vi "Read Message.vi"(8 "error in (no error)":errorcluster, 10 "Bytes to read":i32, 11 "TCP Listener in":refnum<class "TCP Listener.lvclass">) -> (0 "error out":errorcluster, 2 "Message string":string, 3 "TCP Listener out":refnum<class "TCP Listener.lvclass">)   [LabVIEW 2026, in "TALOS.lvlib" / "TCP Listener.lvlib" / "TCP Listener.lvclass"]
uses:
  TCP Listener.lvclass
  TCP Listener.lvclass/TCP Listener.ctl
  Support VIs/Global Constants.vi
  TALOS.lvlib
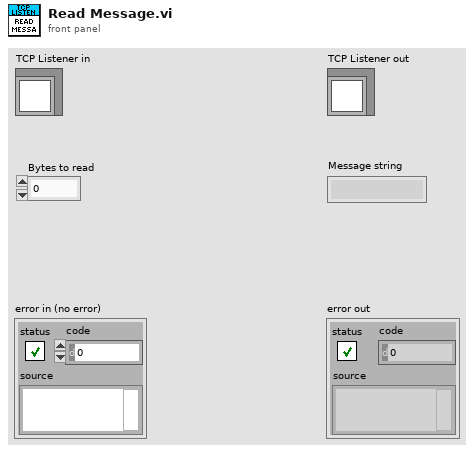
[diagram p1: front panel]
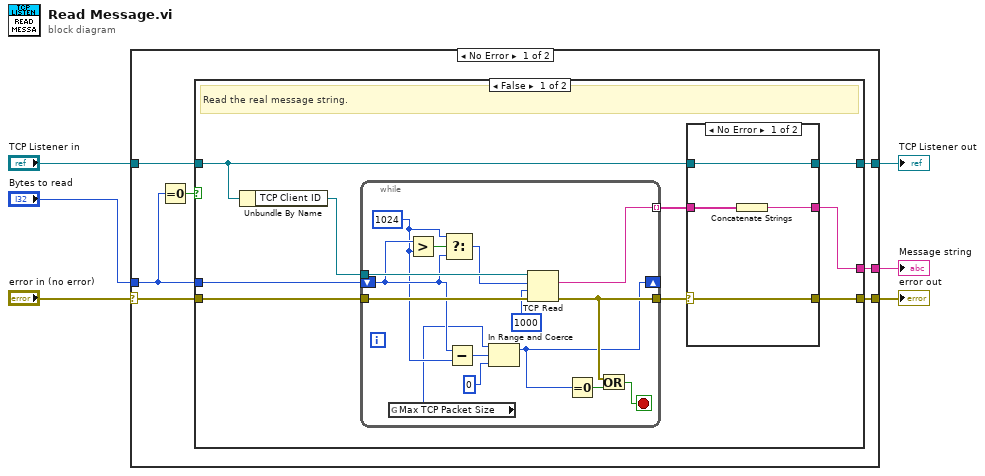
[diagram p0: block diagram]
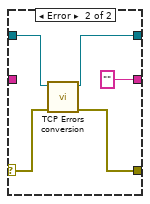
[diagram p2: hidden frame]
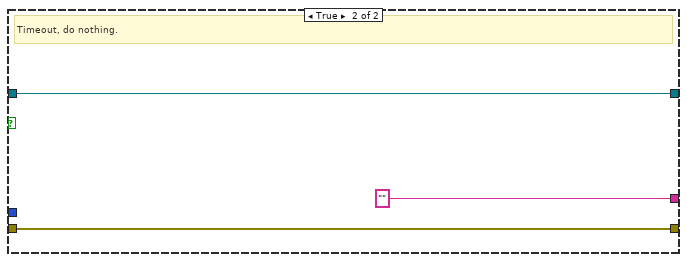
[diagram p3: hidden frame]
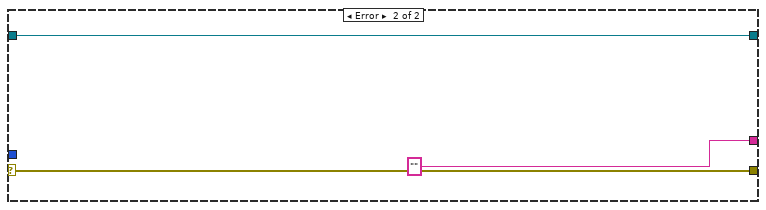
[diagram p4: hidden frame]
diagram:
  n1 = case shown="No Error" "error in (no error)" {
    selector: "error in (no error)" -> [w13 w52]
    tunnel: [w10 w52] -> w5
    tunnel: [w11 w51] -> w3
    tunnel: "TCP Listener in" -> [w12 w51]
    tunnel: "Bytes to read" -> [w7 _]
    tunnel: [w9 ""] -> w1
    frame No Error {
      n2 = Equal To 0?(x=w7) -> (x = 0?=w8:bool)
      n3 = case shown="False" w8 {
        tunnel: w7 -> [w21 _]
        tunnel: w13 -> [w20 w47]
        tunnel: w12 -> [w19 w49]
        tunnel: [w16 w49] -> w11
        tunnel: [w15 w47] -> w10
        tunnel: [w14 "" ("data out")] -> w9
        frame False {
          # "Read the real message string."
          n4 = Unbundle By Name(w19) -> ("TCP Client ID"=w22:refnum<k5>)
          n5 = while {
            tunnel: w22 -> [w37]
            tunnel: [w35] -> w17 mode=indexing
            tunnel: w20 -> [w36]
            tunnel: [w25] -> w18
            shift-right: [w24] -> _
            shift-left: w21 -> [w31]
            stop <- w27 stop-if-true
            w30 = 1024 ("timeout ms (25000)")
            n6 = global read "Global Constants.vi" "Max TCP Packet Size"() -> (w23:i32)
            n7 = Greater?(x=w31, y=w30) -> (0:w33:bool)
            n8 = Select(t=w30, s=w33, f=w31) -> (s? t:f=w32:i32)
            n9 = Subtract(x=w31, y=w30) -> (x-y=w29:i32)
            n10 = In Range and Coerce(upper limit=w23, x=w29, lower limit=0) -> (coerced(x)=w24:i32)  [unwired: 1 out]
            n11 = TCP Read(connection ID=w37, bytes to read=w32, error in (no error)=w36, 9:1000 ("timeout ms (25000)")) -> (data out=w35:string, error out=w25:errorcluster)  [unwired: 1 in, 1 out]
            n12 = Equal To 0?(x=w24) -> (x = 0?=w26:bool)
            n13 = Or(x=w25, y=w26) -> (x .or. y?=w27:bool)
          }
          n14 = case shown="No Error" w18 {
            selector: w18 -> [w40 w45]
            tunnel: w19 -> [w39 w46]
            tunnel: w17 -> [w41 _]
            tunnel: [w39 w44] -> w16
            tunnel: [w40 w43] -> w15
            tunnel: [w38 ""] -> w14
            frame No Error {
              n15 = Concatenate Strings(w41) -> (w38:string)
            }
            frame Error {
              n16 = call-dynamic "TCP Errors conversion.vi"("error in (no error)"=w45, "TCP Listener in"=w46) -> ("error out"=w43:errorcluster, "TCP Listener out"=w44:refnum<class "TCP Listener.lvclass">)  [unwired: 8 in]
            }
          }
        }
        frame True {
          # "Timeout, do nothing."
        }
      }
    }
    frame Error {
    }
  }
  "error out" <- w5
  "TCP Listener out" <- w3
  "Message string" <- w1
